vi "Send Gmail - Multiple Attach (SubVI).vi"(0 "Program/Location Name":string="Program", 2 "Send Email Button":bool, 5 "Test Operator (First Last)":string="User", 7 "Test Name (Subject)":string, 9 "Test Description (Body)":string, 11 "Error IN":errorcluster, 12 "Alternate Email":string, 13 "Send Email Signal (Event)":bool, 14 "Attachment Path(s)":path[](array[path])) -> (4 "Email Sent?":bool, 8 "Last Sent Time":timestamp format="%<%I:%M:%S %p\n%x>T", 15 "Email Error":errorcluster)   [LabVIEW 2012]
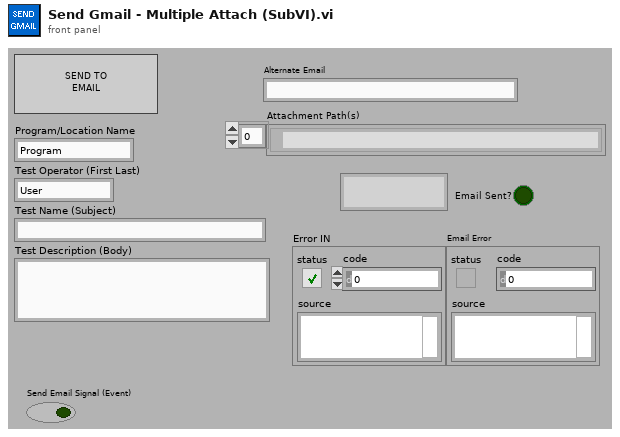
[diagram p1: front panel]
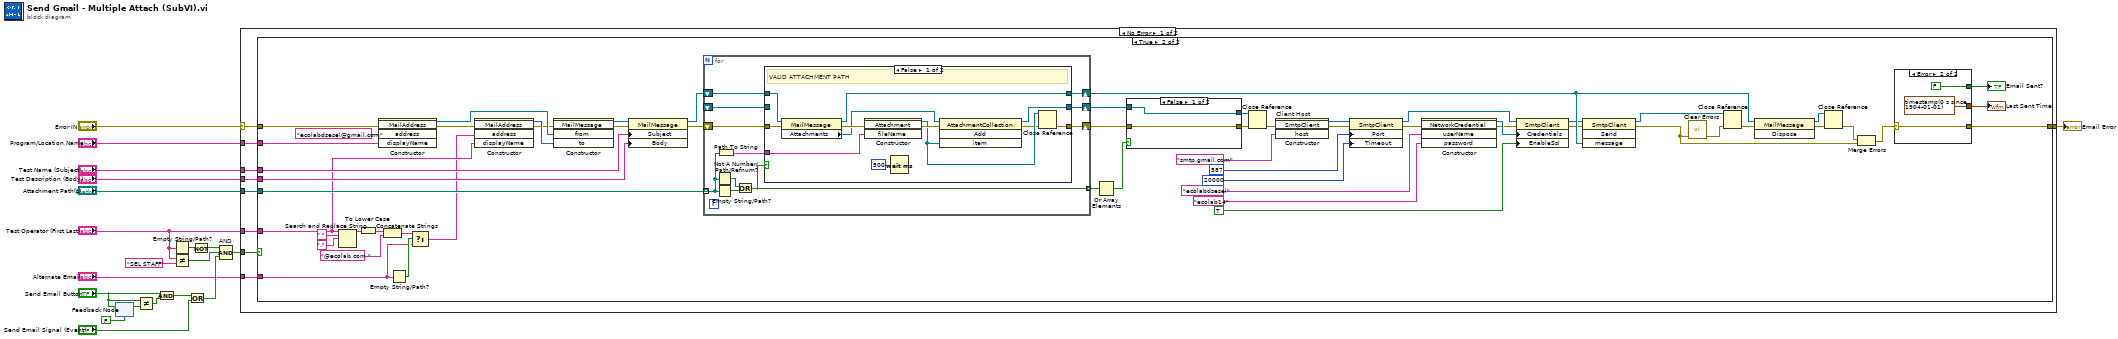
[diagram p0: block diagram]
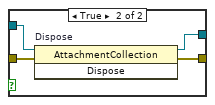
[diagram p3: hidden frame]
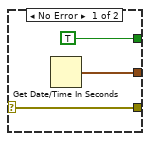
[diagram p5: hidden frame]
diagram:
  n1 = feedback-in #1("Send Email Button") -> ()
  n2 = feedback #1(FALSE) -> (w17:bool)
  n3 = Not Equal?(x="Send Email Button", y=w17) -> (x != y?=w16:bool)
  n4 = And(x="Send Email Button", y=w16) -> (x .and. y?=w7:bool)
  n5 = Empty String/Path?(string/path="Test Operator (First Last)") -> (empty?=w13:bool)
  n6 = Not Equal?(x="Test Operator (First Last)", y="SEL STAFF") -> (x != y?=w11:bool)
  n7 = Or(x=w7, y="Send Email Signal (Event)") -> (x .or. y?=w5:bool)
  n8 = Not(x=w13) -> (.not. x?=w12:bool)
  n9 = Compound Arithmetic op=AND "AND"(w12, w11, w5) -> (w10:bool)
  n10 = case shown="No Error" "Error IN" {
    selector: "Error IN" -> [w22 w126]
    tunnel: "Program/Location Name" -> [w29 _]
    tunnel: "Test Name (Subject)" -> [w28 _]
    tunnel: "Test Description (Body)" -> [w27 _]
    tunnel: "Test Operator (First Last)" -> [w26 _]
    tunnel: w10 -> [w25 _]
    tunnel: "Attachment Path(s)" -> [w24 _]
    tunnel: "Alternate Email" -> [w23 _]
    tunnel: [w21 w126] -> w2
    frame No Error {
      n11 = case shown="True" w25 {
        tunnel: w29 -> [_ w87]
        tunnel: w28 -> [_ w86]
        tunnel: w27 -> [_ w82]
        tunnel: w26 -> [_ w76]
        tunnel: w24 -> [_ w85]
        tunnel: w23 -> [_ w36]
        tunnel: w22 -> [w30 w75]
        tunnel: [w30 w74] -> w21
        frame False {
        }
        frame True {
          n12 = Search and Replace String(input string=w76, search string=" ", replace string="." ("replace string (\"\")")) -> (result string=w79:string)  [unwired: 5 in, 3 out]
          n13 = To Lower Case(string=w79) -> (all lower case string=w80:string)
          n14 = constructor class="MailAddress"(error in=w75, "address"="ecolabdsesel@gmail.com" ("Sender's Email Address (eg: jsmith77@gmail.com)"), "displayName"=w87) -> (reference out=w72:refnum<k24>, error out=w54:errorcluster)  [unwired: 2 in, 3 out]
          n15 = Concatenate Strings(w80, "@ecolab.com " ("search string")) -> (w38:string)
          n16 = Empty String/Path?(string/path=w36) -> (empty?=w37:bool)
          n17 = Select(t=w38, s=w37, f=w36) -> (s? t:f=w35:string)
          n18 = constructor class="MailAddress"(error in=w54, "address"=w35, "displayName"=w76) -> (reference out=w73:refnum<k24>, error out=w53:errorcluster)  [unwired: 2 in, 3 out]
          n19 = constructor class="MailMessage"(error in=w53, "from"=w72, "to"=w73) -> (reference out=w62:refnum<k24>, error out=w61:errorcluster)  [unwired: 2 in, 3 out]
          n20 = property class="MailMessage"(reference=w62, error in=w61, "Subject"=w86, "Body"=w82) -> (reference out=w45:refnum<k24>, error out=w44:errorcluster)
          n21 = for {
            tunnel: w85 -> [w101] mode=indexing
            shift-right: [w104] -> w59
            shift-left: _ -> [w95]
            shift-right: [w99] -> w41
            shift-left: w44 -> [w96]
            shift-right: [w97] -> w52
            shift-left: w45 -> [w98]
            tunnel: [w94] -> w43 mode=indexing
            n22 = Not A Number/Path/Refnum?(number/path/refnum=w101) -> (NaN/Path/Refnum?=w102:bool)
            n23 = Empty String/Path?(string/path=w101) -> (empty?=w103:bool)
            n24 = Path To String(path=w101) -> (string=w100:string)
            n25 = Or(x=w102, y=w103) -> (x .or. y?=w94:bool)
            n26 = case shown="False" w94 {
              tunnel: [w116 w117] -> w104
              tunnel: [w105 w118] -> w99
              tunnel: w100 -> [w113 _]
              tunnel: w98 -> [w112 w119]
              tunnel: [w111 w119] -> w97
              tunnel: w96 -> [w110 w118]
              tunnel: w95 -> [_ w117]
              frame False {
                # "VALID ATTACHMENT PATH"
                n27 = property class="MailMessage"(reference=w112, error in=w110) -> (reference out=w111:refnum<k24>, error out=w109:errorcluster, "Attachments"=w108:refnum<k24>)
                n28 = constructor class="Attachment"(error in=w109, "fileName"=w113) -> (reference out=w107:refnum<k24>, error out=w114:errorcluster)  [unwired: 2 in, 2 out]
                n29 = Wait (ms)(milliseconds to wait=u32 500) -> ()  [unwired: 1 out]
                n30 = invoke class="AttachmentCollection" method="Add"(reference=w108, error in=w114, "item"=w107) -> (reference out=w116:refnum<k24>, error out=w106:errorcluster)  [unwired: 1 in, 2 out]
                n31 = Close Reference(reference=w107, error in (no error)=w106) -> (error out=w105:errorcluster)
              }
              frame True {
                # "INVALID ATTACHMENT PATH"
              }
            }
          }
          n32 = Or Array Elements(Boolean array=w43) -> (logical OR=w42:bool)
          n33 = case shown="False" w42 {
            tunnel: w59 -> [w88 w93]
            tunnel: w41 -> [w89 w92]
            tunnel: [w89 w91] -> w56
            tunnel: [w88 w90] -> w55
            frame False {
            }
            frame True {
              n34 = invoke on="Dispose" class="AttachmentCollection" method="Dispose"(reference=w93, error in=w92) -> (reference out=w90:refnum<k24>, error out=w91:errorcluster)  [unwired: 1 in, 1 out]
            }
          }
          n35 = Close Reference(reference=w55, error in (no error)=w56) -> (error out=w40:errorcluster)
          n36 = constructor on="Client Host" class="SmtpClient"(error in=w40, "host"="smtp.gmail.com" ("Outgoing Mail Server (SMTP)")) -> (reference out=w65:refnum<k24>, error out=w63:errorcluster)  [unwired: 2 in, 2 out]
          n37 = property class="SmtpClient"(reference=w65, error in=w63, "Port"=587, "Timeout"=20000) -> (reference out=w64:refnum<k24>, error out=w58:errorcluster)
          n38 = constructor class="NetworkCredential"(error in=w58, "userName"="ecolabdsesel" ("GMAIL Account User ID (eg: jsmity77)"), "password"="ecolab14" ("GMAIL Account Password")) -> (reference out=w66:refnum<k24>, error out=w57:errorcluster)  [unwired: 2 in, 3 out]
          n39 = property class="SmtpClient"(reference=w64, error in=w57, "Credentials"=w66, "EnableSsl"=TRUE ("Enable SSL")) -> (reference out=w49:refnum<k24>, error out=w48:errorcluster)
          n40 = invoke class="SmtpClient" method="Send"(reference=w49, error in=w48, "message"=w52) -> (reference out=w60:refnum<k24>, error out=w32:errorcluster)  [unwired: 1 in, 2 out]
          n41 = call <vilib>:"Clear Errors.vi"("error in (no error)"=w32) -> ("error out"=w34:errorcluster)  [unwired: 6 in]
          n42 = Close Reference(reference=w60, error in (no error)=w34) -> (error out=w39:errorcluster)
          n43 = invoke class="MailMessage" method="Dispose"(reference=w52, error in=w39) -> (reference out=w51:refnum<k24>, error out=w46:errorcluster)  [unwired: 1 in, 1 out]
          n44 = Close Reference(reference=w51, error in (no error)=w46) -> (error out=w33:errorcluster)
          n45 = Merge Errors(w33, w32) -> (w31:errorcluster)
          n46 = case shown="Error" w31 {
            selector: w31 -> [w120 w123]
            tunnel: [TRUE FALSE] -> w83
            tunnel: [w121 timestamp(0 s since 1904-01-01) ("seconds since 1Jan1904")] -> w84
            tunnel: [w120 w123] -> w74
            frame No Error {
              n47 = Get Date/Time In Seconds() -> (seconds since 1Jan1904=w121:timestamp)
            }
            frame Error {
            }
          }
          "Last Sent Time" <- w84
          "Email Sent?" <- w83
        }
      }
    }
    frame Error {
    }
  }
  "Email Error" <- w2
